vi "Read Image Buffer.vi"(0 "buffHandle IN":u32, 1 "Image Reference IN":T2, 3 "Camera Image Info":T1={"Frame"=0, "Sensor Height"=0, "Sensor Width"=0, "ROI Height"=0, "ROI Width"=0, "ROI Enable?"=FALSE, "Bit per Pixel"=0, "Binning factor"=1} {"Binning factor" min=1}, 5 "Error IN":errorcluster, 10 "Pixel format":T3 items=["Mono8"=257, "Mono10"=258, "Mono12"=259]) -> (14 "Image Reference OUT":T2, 16 "frame index":i32, 18 "Array OUT":u16[](array[numeric]), 19 "Error OUT":errorcluster)   [LabVIEW 2020]
uses:
  VPD Controls/VPD Pixel format.ctl
  <vilib>/vision/Image Controls.llb/IMAQ Image.ctl
  Cameras/Camera Controls/Camera IMAQ Key Info.ctl
  Desktop/Vision Point LabVIEW/KYFGLib_lv.lvlib
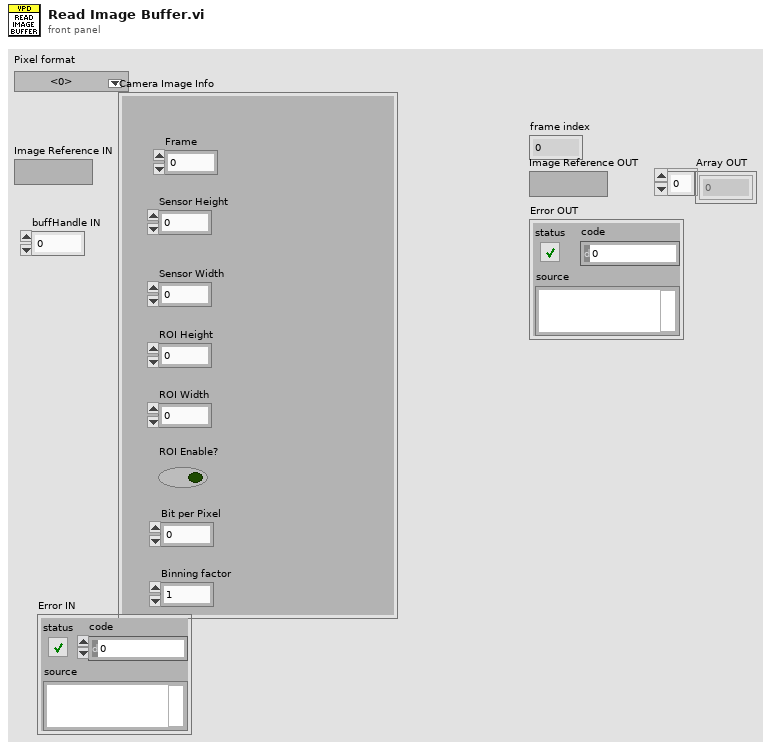
[diagram p1: front panel]
types:
  T1 = typedef "Camera IMAQ Key Info.ctl" = cluster{"Frame":u32, "Sensor Height":i32, "Sensor Width":i32, "ROI Height":i32, "ROI Width":i32, "ROI Enable?":bool, "Bit per Pixel":u8, "Binning factor":i32}
  T2 = typedef "IMAQ Image.ctl" = refnum<image>
  T3 = typedef "VPD Pixel format.ctl" = i64
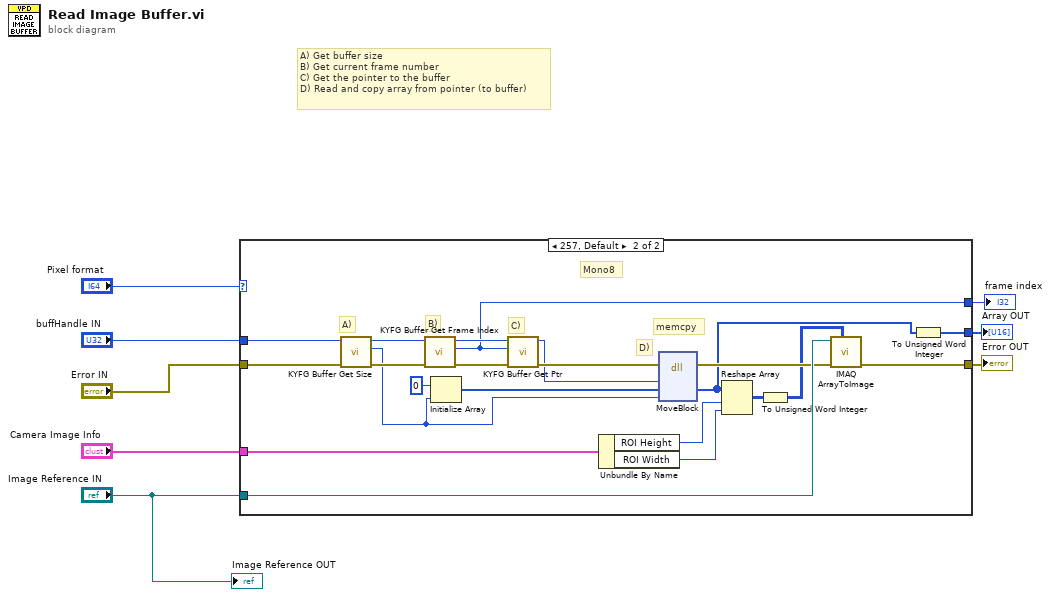
[diagram p0: block diagram]
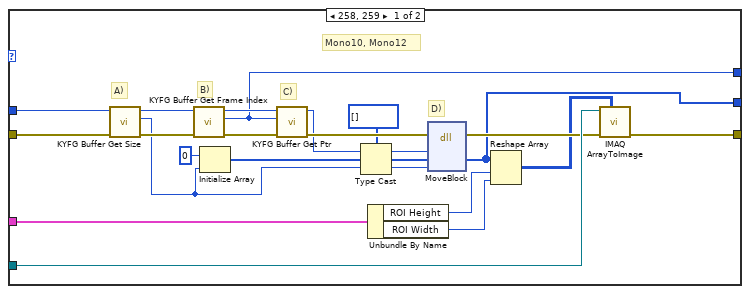
[diagram p2: hidden frame]
diagram:
  # "A) Get buffer size\nB) Get current frame number\nC) Get the pointer to the buffer\nD) Read and copy array from pointer (to buffer)"
  n1 = case shown="257, Default" "Pixel format" {
    tunnel: [w11 w35] -> w3
    tunnel: [w18 w43] -> w8
    tunnel: "buffHandle IN" -> [w19 w44]
    tunnel: "Image Reference IN" -> [w17 w41]
    tunnel: "Camera Image Info" -> [w16 w40]
    tunnel: "Error IN" -> [w13 w37]
    tunnel: [w9 w32] -> w1
    frame 258, 259 {
      # "D)"
      # "C)"
      # "B)"
      # "A)"
      # "Mono10, Mono12"
      n2 = call "KYFG Buffer Get Size.vi"("error in (no error)"=w13, "buffHandle"=w19) -> ("error out"=w30:errorcluster, "buffer size"=w20:i32, "buffHandle out"=w28:u32)  [unwired: 7 in]
      n3 = call "KYFG Buffer Get Frame Index.vi"("error in (no error)"=w30, "buffHandle"=w28) -> ("error out"=w29:errorcluster, "frame index"=w18:i32, "buffHandle out"=w27:u32)  [unwired: 7 in]
      n4 = Initialize Array(u8 0 ("I32"), w20) -> (w23:u8[])
      n5 = call "KYFG Buffer Get Ptr.vi"("error in (no error)"=w29, "frame"=w18, "buffHandle"=w27) -> ("error out"=w25:errorcluster, "buffer data"=w24:u64)  [unwired: 7 in]
      n6 = Type Cast(type=u16[] [] ("initialized array"), x=w23) -> (*(type *) &x=w22:u16[])
      n7 = Unbundle By Name(w16) -> ("ROI Height"=w15:i32, "ROI Width"=w14:i32)
      n8 = dll-call lib="LabVIEW" fn="MoveBlock"(error in=w25, "src"=w24, "dst"=w22, "size"=w20) -> (error out=w12:errorcluster, "dst"=w9:u16[])  [unwired: 5 in, 1 out]
      n9 = Reshape Array(w9, w15, w14) -> (w10:u16[][])
      n10 = call "IMAQ ArrayToImage"("Image Pixels (U16)"=w10, "error in (no error)"=w12, "Image"=w17) -> ("error out"=w11:errorcluster)  [unwired: 7 in, 1 out]
    }
    frame 257, Default {
      # "D)"
      # "C)"
      # "B)"
      # "A)"
      # "Mono8"
      # "memcpy"
      n11 = call "KYFG Buffer Get Size.vi"("error in (no error)"=w37, "buffHandle"=w44) -> ("error out"=w52:errorcluster, "buffer size"=w45:i32, "buffHandle out"=w50:u32)  [unwired: 7 in]
      n12 = call "KYFG Buffer Get Frame Index.vi"("error in (no error)"=w52, "buffHandle"=w50) -> ("error out"=w51:errorcluster, "frame index"=w43:i32, "buffHandle out"=w49:u32)  [unwired: 7 in]
      n13 = Initialize Array(u8 0 ("I32"), w45) -> (w42:u8[])
      n14 = call "KYFG Buffer Get Ptr.vi"("error in (no error)"=w51, "frame"=w43, "buffHandle"=w49) -> ("error out"=w47:errorcluster, "buffer data"=w46:u64)  [unwired: 7 in]
      n15 = Unbundle By Name(w40) -> ("ROI Height"=w39:i32, "ROI Width"=w38:i32)
      n16 = dll-call lib="LabVIEW" fn="MoveBlock"(error in=w47, "src"=w46, "dst"=w42, "size"=w45) -> (error out=w36:errorcluster, "dst"=w31:u8[])  [unwired: 5 in, 1 out]
      n17 = Reshape Array(w31, w39, w38) -> (w34:u8[][])
      n18 = To Unsigned Word Integer(number=w34) -> (unsigned 16bit integer=w33:u16[][])
      n19 = call "IMAQ ArrayToImage"("Image Pixels (U16)"=w33, "error in (no error)"=w36, "Image"=w41) -> ("error out"=w35:errorcluster)  [unwired: 7 in, 1 out]
      n20 = To Unsigned Word Integer(number=w31) -> (unsigned 16bit integer=w32:u16[])
    }
  }
  "frame index" <- w8
  "Error OUT" <- w3
  "Array OUT" <- w1
  "Image Reference OUT" <- "Image Reference IN"
